vi "FTW-SQLite-OpenConnection-Path.vi"(5 "Database Filepath":path, 7 "Access Mode":T1, 11 "error in":errorcluster) -> (4 "SQLite Connector":refnum<class "FTW-SQLite-Connector.lvclass">, 15 "error out":errorcluster)   [LabVIEW 2013, in "FTW-SQLite-Connector.lvclass"]
uses:
  FTW-SQLite-Connector.lvclass
  FTW-SQLite-AccessMode.ctl
  FTW-SQLite-DatabaseType.ctl
panel:
  # "Inputs"
  # "Outputs"
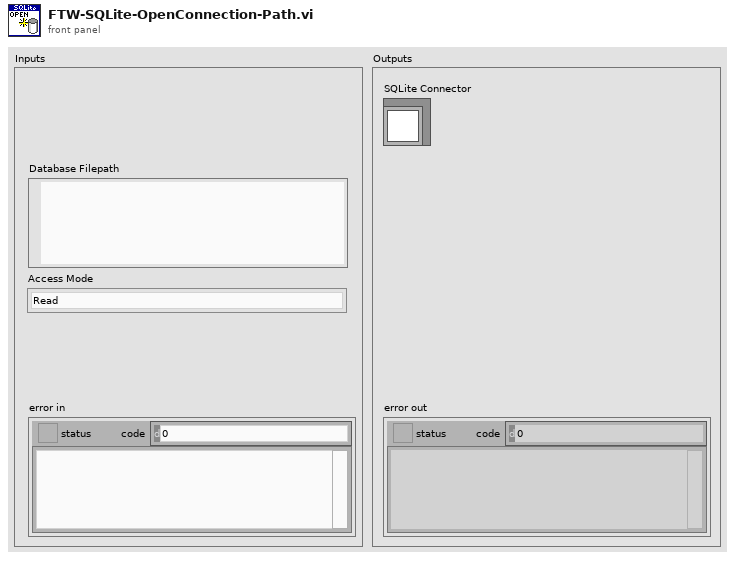
[diagram p1: front panel]
types:
  T1 = typedef "FTW-SQLite-Connector.lvclass/FTW-SQLite-AccessMode.ctl" = enum16{"Read", "Read/Write", "Read/Write/Create"}
  T2 = typedef "FTW-SQLite-Connector.lvclass/FTW-SQLite-DatabaseType.ctl" = enum16{"Disk", "Memory"}
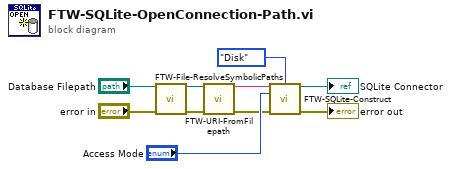
[diagram p0: block diagram]
diagram:
  n1 = call "FTW-File-ResolveSymbolicPaths.vi"("Unresolved Path"="Database Filepath", "error in"="error in") -> ("Resolved Path"=w3:path, "error out"=w1:errorcluster)  [unwired: 12 in]
  n2 = call "FTW-URI-FromFilepath.vi"("Path"=w3, "error in"=w1) -> ("URI"=w6:string, "error out"=w7:errorcluster)  [unwired: 12 in]
  n3 = call "FTW-SQLite-Construct.vi"("Database URI"=w6, "Database Type"=FTW-SQLite-DatabaseType."Disk", "Access Mode"="Access Mode", "error in"=w7) -> ("SQLite Connector"=→"SQLite Connector":refnum<class "FTW-SQLite-Connector.lvclass">, "error out"=→"error out":errorcluster)  [unwired: 9 in, 1 out]
